vi "WS1050 16 DUT VSA-CV Sweep HD_Cycling_Ver1.3.vi"() -> ()   [LabVIEW 2012]
uses:
  WS_VCAP Driver 024/Source/WSVCAP Shell/Type Defs/WSVCAP SHL I2C DUT Mask Mode Enum.ctl
  <vilib>/Utility/file.llb/Read From Spreadsheet File (DBL).vi
panel:
  out "VISA resource name out":refnum<visa-resource-name>="GPIB0::3::INSTR"
  out "date string":string="5/19/2014"
  out "PS1 Out":refnum<visa-resource-name>
  out "Ke2000 Out":refnum<visa-resource-name>="GPIB0::9::INSTR"
  in  "Tab Control":enum32{"Inst Control", "Data Output", "Graphs"}(tab)
  in  "Bank to HD":u16(ring)=5 items=["All OFF", "All ON", "Bank_C1", "Bank_C2", "Bank_C3", "F12+B1"]
  out "AD7747 Values":string[][](table)
  in  "Lot#":string="4NEMB"
  in  "Wafer#":string="20-EB"
  in  "File Name":string="HD_4NEMB_25_EB_65C_44V_100DC_BRD2_150916_1"
  in  "TMN DC\\CAP Data Log File Path":path=path "C:/WS1050 16 DUT Data"
  in  "SN":string[](array[string])=["1", "2", "3", "4", "5", "6", "7", "8", "9", "10", "11", "12", "13", "14", "15", "16"]
  in  "Test Program":string="WS1050 16 DUT VSA_CV Sweep HD_Cycling Ver1.3"
  out "Current Date":string="8/28/2014"
  out "Current Time":string="0950"
  in  "Start Date":string="4/24/2014"
  in  "Start Time":string="1542"
  in  "Comment":string="CV Sweep"
  in  "OK Button":bool
  in  "Calibration":bool
  in  "Control Setting":bool
  in  "CP Setting":i32(ring) items=["CP OFF", "CP ON", "CP 35V", "CP 40V", "CP 44V", "CP 50V", "DVA OFF", "DVA ON", "Reg1 ON", "Reg1 OFF", "Reg2 ON", "Reg2 OFF", "Reg3 ON", "Reg3 OFF"]
  in  "VDD(V)":dbl=3.3 format="%.3g"
  in  "Meas Clock Rate (Hz)":dbl=1000000.0 caption="Meas Speed" format="%.1p Hz"
  out "AR  Measurent(Hz)":dbl
  in  "PS1 Source":refnum<visa-resource-name>="GPIB0::5::INSTR"
  in  "Ke2000":refnum<visa-resource-name>="GPIB0::9::INSTR"
  out "Simulate FPGA":bool
  out "Online":bool
  in  "Ke2400":refnum<visa-resource-name>="GPIB0::3::INSTR"
  in  "Initialize AD7747":bool
  in  "DUT Mask Mode":T1=enum."All"
  in  "RFFE Slave Address":u8=7 caption="Slave Address" format="0x%02x"
  out "Activity Log":string="05/19/2014 -- 12:24:35.853::WSVCAP::APP::Application Started\n05/19/2014 -- 12:24:37.606::WSVCAP::WSVCAP SHL::WR I2C-REG:0x0A;MASK:0xFFFFFFFFFFFF;C1 DATA:22:22:22:22:22:22:22:22:22:22:22:22:22:22:22:22;C2 DATA:22:22:22:22:22:22:22:22:22:22:22:22:22:22:22:22;C3 DATA:22:22:22:22:22:22:22:22:22:22:22:22:22:22:22:22\r\n05/19/2014 -- 12:24:37.773::WSVCAP::WSVCAP SHL::WR I2C-ST:0,0,4,1\r\n05/19/2014 -- 12:24:37.903::WSVCAP::WSVCAP SHL::RD I2C-BYTES:4;ADD:0x00;MASK:0xFFFFFFFFFFFF\r\n05/19/2014 -- 12:24:38.045::WSVCAP::WSVCAP SHL::RD I2C:C1 DATA:2:2:2:2:2:2:2:2:2:2:2:2:2:2:2:2|A7:A9:AA:82:82:7F:82:81:82:81:83:82:81:82:82:81|46:36:BB:88:44:A3:E9:2B:32:20:ED:25:BB:3D:68:B|2C:6A:EB:A7:22:56:FE:CC:36:82:D7:B0:3B:48:F9:CC;C2 DATA:2:2:2:2:2:2:2:2:2:2:2:2:2:2:2:2|94:94:94:80:80:80:80:80:81:7E:7E:81:80:7E:80:80|47:33:15:82:62:B:E8:1C:D7:C3:7D:41:7C:B7:4C:2A|C4:B4:AE:8:1E:D1:4E:37:11:C0:6F:63:42:9D:63:B5;C3 DATA:2:2:2:2:2:2:2:2:2:2:2:2:2:2:2:2|95:95:95:81:81:7E:81:80:84:7D:80:83:81:7E:7F:80|AB:C4:14:B5:7B:52:DF:C9:79:5D:5F:30:99:31:1E:F4|6E:5C:F7:A8:C3:EB:7B:EF:33:92:89:77:4D:67:75:DD;STATUS:0:0:4:0\r\n05/19/2014 -- 12:24:38.046::WSVCAP::WSVCAP SHL::WR I2C-REG:0x0A;MASK:0xFFFFFFFFFFFF;C1 DATA:22:22:22:22:22:22:22:22:22:22:22:22:22:22:22:22;C2 DATA:22:22:22:22:22:22:22:22:22:22:22:22:22:22:22:22;C3 DATA:22:22:22:22:22:22:22:22:22:22:22:22:22:22:22:22\r\n05/19/2014 -- 12:24:38.089::WSVCAP::WSVCAP SHL::WR I2C-ST:0,0,4,1\r\n05/19/2014 -- 12:24:38.219::WSVCAP::WSVCAP SHL::RD I2C-BYTES:4;ADD:0x00;MASK:0xFFFFFFFFFFFF\r\n05/19/2014 -- 12:24:38.362::WSVCAP::WSVCAP SHL::RD I2C:C1 DATA:2:2:2:2:2:2:2:2:2:2:2:2:2:2:2:2|A7:AB:AA:82:82:82:83:83:82:82:82:82:7F:82:82:81|4B:32:96:83:3E:61:43:17:25:62:AB:4D:A2:40:2E:5|3C:76:2B:B4:EE:E4:A9:1A:AA:A:26:C7:21:2E:87:5B;C2 DATA:2:2:2:2:2:2:2:2:2:2:2:2:2:2:2:2|94:94:94:80:80:80:80:80:80:7F:80:81:80:80:7F:80|4A:32:19:7D:19:6C:79:46:61:7F:4B:B8:A5:30:F3:14|B4:70:A:8C:9C:DC:43:FA:1E:A:C6:21:A:A9:13:F3;C3 DATA:2:2:2:2:2:2:2:2:2:2:2:2:2:2:2:2|95:97:94:81:80:81:82:81:80:7E:81:84:7F:81:80:80|B2:32:D0:A7:9E:4C:AB:D4:EE:D9:F0:82:B7:91:7:FF|C1:91:B6:3D:D8:E:1B:4F:9F:6A:F1:6C:E7:3F:7:BA;STATUS:0:0:4:0\r\n05/19/2014 -- 12:24:38.364::WSVCAP::WSVCAP SHL::WR I2C-REG:0x0A;MASK:0xFFFFFFFFFFFF;C1 DATA:22:22:22:22:22:22:22:22:22:22:22:22:22:22:22:22;C2 DATA:22:22:22:22:22:22:22:22:22:22:22:22:22:22:22:22;C3 DATA:22:22:22:22:22:22:22:22:22:22:22:22:22:22:22:22\r\n05/19/2014 -- 12:24:38.406::WSVCAP::WSVCAP SHL::WR I2C-ST:0,0,4,1\r\n05/19/2014 -- 12:24:38.536::WSVCAP::WSVCAP SHL::RD I2C-BYTES:4;ADD:0x00;MASK:0xFFFFFFFFFFFF\r\n05/19/2014 -- 12:24:38.678::WSVCAP::WSVCAP SHL::RD I2C:C1 DATA:2:2:2:2:2:2:2:2:2:2:2:2:2:2:2:2|A7:A9:AB:82:82:81:82:82:82:82:82:82:82:82:82:81|46:71:4C:87:43:3D:7F:FC:25:4F:8E:54:97:3E:60:8C|AA:F4:1F:B5:CE:43:1F:36:9:87:9C:78:86:5:B6:8E;C2 DATA:2:2:2:2:2:2:2:2:2:2:2:2:2:2:2:2|94:94:94:80:7F:7F:80:80:80:80:80:81:80:80:80:80|49:36:18:7D:6E:C5:E4:3C:81:2E:41:D3:75:71:E3:72|E8:D3:E6:D1:E0:48:AE:D4:54:D:E8:8E:B4:41:68:4;C3 DATA:2:2:2:2:2:2:2:2:2:2:2:2:2:2:2:2|95:95:95:81:7F:7F:81:81:81:81:81:84:81:81:82:81|B3:F5:90:AB:82:69:7B:93:D0:77:E8:D5:E8:8C:84:E8|B9:AC:EE:2B:B6:71:8F:4A:74:31:56:BB:8A:B7:A0:C8;STATUS:0:0:4:0\r\n05/19/2014 -- 12:24:38.681::WSVCAP::WSVCAP SHL::WR I2C-REG:0x0A;MASK:0xFFFFFFFFFFFF;C1 DATA:22:22:22:22:22:22:22:22:22:22:22:22:22:22:22:22;C2 DATA:22:22:22:22:22:22:22:22:22:22:22:22:22:22:22:22;C3 DATA:22:22:22:22:22:22:22:22:22:22:22:22:22:22:22:22\r\n05/19/2014 -- 12:24:38.723::WSVCAP::WSVCAP SHL::WR I2C-ST:0,0,4,1\r\n05/19/2014 -- 12:24:38.854::WSVCAP::WSVCAP SHL::RD I2C-BYTES:4;ADD:0x00;MASK:0xFFFFFFFFFFFF\r\n05/19/2014 -- 12:24:38.996::WSVCAP::WSVCAP SHL::RD I2C:C1 DATA:2:2:2:2:2:2:2:2:2:2:2:2:2:2:2:2|A7:A9:AA:82:82:7F:83:81:82:81:84:82:7F:82:7F:82|43:FB:E:7F:3C:AD:35:35:26:A2:6C:21:4B:3D:8:6|63:9A:E1:F3:95:32:91:42:90:3C:78:1F:5C:D7:5F:D8;C2 DATA:2:2:2:2:2:2:2:2:2:2:2:2:2:2:2:2|94:94:94:80:80:80:80:80:81:80:7E:81:80:7E:7F:80|48:36:18:7F:5E:3D:69:83:DE:AE:A1:9E:31:AE:BB:96|15:A0:44:17:13:FD:CC:C8:6D:B2:EF:A7:C:C7:3B:F;C3 DATA:2:2:2:2:2:2:2:2:2:2:2:2:2:2:2:2|95:96:94:81:81:7E:82:80:84:80:80:84:7F:7E:7D:82|AD:3B:6D:A9:7C:57:9D:F5:7A:96:23:5C:36:2D:ED:5A|CD:46:DB:3B:C7:BD:70:60:33:B8:B:F7:63:A:51:4D;STATUS:0:0:4:0\r\n05/19/2014 -- 12:24:38.998::WSVCAP::WSVCAP SHL::WR I2C-REG:0x0A;MASK:0xFFFFFFFFFFFF;C1 DATA:22:22:22:22:22:22:22:22:22:22:22:22:22:22:22:22;C2 DATA:22:22:22:22:22:22:22:22:22:22:22:22:22:22:22:22;C3 DATA:22:22:22:22:22:22:22:22:22:22:22:22:22:22:22:22\r\n05/19/2014 -- 12:24:39.040::WSVCAP::WSVCAP SHL::WR I2C-ST:0,0,4,1\r\n05/19/2014 -- 12:24:39.170::WSVCAP::WSVCAP SHL::RD I2C-BYTES:4;ADD:0x00;MASK:0xFFFFFFFFFFFF\r\n05/19/2014 -- 12:24:39.311::WSVCAP::WSVCAP SHL::RD I2C:C1 DATA:2:2:2:2:2:2:2:2:2:2:2:2:2:2:2:2|A7:AA:AB:82:82:81:82:81:82:81:82:82:82:82:7F:82|44:F1:90:87:45:44:C8:2C:2C:F1:FC:1B:94:3B:3C:75|4A:49:95:19:99:73:64:3:23:24:F3:A2:5E:7F:C4:B6;C2 DATA:2:2:2:2:2:2:2:2:2:2:2:2:2:2:2:2|94:94:94:80:80:80:80:7F:80:80:7E:80:80:7E:7F:80|4C:36:17:7D:A8:9F:DE:C7:53:6D:8A:F4:41:A5:C6:E0|90:2E:24:C:D9:22:E4:76:3B:40:1D:53:33:B1:3E:4D;C3 DATA:2:2:2:2:2:2:2:2:2:2:2:2:2:2:2:2|95:97:95:81:81:7F:81:80:80:81:7F:82:81:7E:7D:82|AE:2B:A7:AB:CC:CD:A4:38:FD:17:80:F2:92:2D:45:C4|76:E5:D:B9:AD:B5:BA:8D:28:32:9E:42:B7:20:4A:D9;STATUS:0:0:4:0\r\n05/19/2014 -- 12:24:39.313::WSVCAP::WSVCAP SHL::WR I2C-REG:0x0A;MASK:0xFFFFFFFFFFFF;C1 DATA:22:22:22:22:22:22:22:22:22:22:22:22:22:22:22:22;C2 DATA:22:22:22:22:22:22:22:22:22:22:22:22:22:22:22:22;C3 DATA:22:22:22:22:22:22:22:22:22:22:22:22:22:22:22:22\r\n05/19/2014 -- 12:24:39.355::WSVCAP::WSVCAP SHL::WR I2C-ST:0,0,4,1\r\n05/19/2014 -- 12:24:39.486::WSVCAP::WSVCAP SHL::RD I2C-BYTES:4;ADD:0x00;MASK:0xFFFFFFFFFFFF\r\n05/19/2014 -- 12:24:39.628::WSVCAP::WSVCAP SHL::RD I2C:C1 DATA:2:2:2:2:2:2:2:2:2:2:2:2:2:2:2:2|A7:A9:AA:82:82:82:83:82:82:82:82:82:7F:82:7F:82|47:18:E4:87:3E:E7:6:65:25:92:37:38:A8:3E:89:85|7C:A7:7:2B:A3:7A:EC:EF:89:ED:F4:D3:D8:BC:3A:F5;C2 DATA:2:2:2:2:2:2:2:2:2:2:2:2:2:2:2:2|94:94:94:80:7F:80:80:7F:81:80:7E:80:80:80:81:80|49:37:17:80:76:25:6A:F8:DF:55:97:4D:B8:5B:2B:B1|13:E3:9A:3E:1A:2D:4F:B6:DB:E9:61:FA:8B:D6:9:CC;C3 DATA:2:2:2:2:2:2:2:2:2:2:2:2:2:2:2:2|95:95:95:81:7F:80:82:81:84:80:7F:81:80:81:7F:82|AF:93:3B:AF:5B:11:82:E4:7E:C3:2D:72:9:96:D9:A|DB:96:F2:10:5F:64:9A:C6:98:12:27:7D:10:D3:20:D9;STATUS:0:0:4:0\r\n05/19/2014 -- 12:24:40.132::WSVCAP::WSVCAP SHL::CLOSE\r\n"
  in  "C1 Cap DAC":u8=128 caption="B Data In" format="0x%02x"
  in  "C2 Cap DAC":u8=128 caption="B Data In" format="0x%02x"
  in  "C3 Cap DAC":u8=128 caption="B Data In" format="0x%02x"
  out "IDD Brd(uA)":string
  in  "VSA_IDD(A)":dbl=0.1
  in  "Stress Voltage(V)":dbl
  in  "Reset PS":bool
  in  "HD/Cycling":bool
  in  "Cyc Clock Rate (Hz)":dbl=5000000.0 caption="Cycle Speed" format="%.1p Hz"
  in  "Bank to Cycle":u16(ring)=1 items=["Cycle All", "Cycle F12+S1", "Cycle All - F12"]
  in  "Set Delay":dbl[](array[numeric])=[1.8e-05, 1.8e-05, 1.8e-05] min=0.0 max=0.5 format="%#.0p s"
  in  "CP Freq":u16(ring)=3 items=["000", "001", "010", "011", "100", "101", "110", "111"]
  in  "CP to HD/Cycle":i32(ring)=4 items=["CP HDC 35V", "CP HDC 40.25V", "CP HDC 27.5V", "CP HDC 30.5V", "CP HDC 44V", "CP HDC 50V"]
  in  "Cycle Freq(KHz)":dbl
  in  "RP will be\nFrom Lookup Table":bool
  out "STATUS":string="Idle...."
  in  "stop":bool
  out "C1 Min_T0":string[](array[string])
  out "CAP_Value(pF)":string[][](array[string])
  out "C3 Min_T0":string[](array[string])
  out "C2 Min_T0":string[](array[string])
  in  "Abort":bool
  out "error out 2":errorcluster
  in  "Set Stress to\nComplete(Cyc/Min)":u64=8100
  out "Verify Test Condition":string[](array[string])
  out "CMin+VCAP":string[][](table)
  out "Verify Drivers to Stress":string[](array[string])
  out "Cycle Count":u64 min=1 max=4 step=1
  out "Stress \nCompleted(Min)":u64
  out "Previous Time":string="12:20:26 PM"
  out "Delta CAP_T0(pF)":dbl[][](array[numeric])
  out "Delta CAP_Tc(pF)":dbl[][](array[numeric])
  in  "error in (no error)":errorcluster
  out "error out":errorcluster
  out "CP_IDD(uA)":string
  # "Company:  WiSpry Inc 20 Fairbanks \nSte 198 Irvine CA 92618\n\nAuthor:  Andy V Tran\nCreated:  01/13/2016\nLabVIEW 2012 Pro\nTP:  WS1050 16 DUT VSA_CV Sweep HD_Cycling Ver1.3\nFPGA Version: WS_VCAP Driver 024"
  # "Note:  Ver1.0 is a original version.\n\n1.  Two look up tables, \n      a.  1st is for Stress\n      b.  2nd is for Voltage sweep\n\nVer1.1\n\n1.  No Voltage to CAP Head for initial read point\n\nVer1.2\n\n1.  Add CP Freq\n\nVer1.3\n\n1.  Add Cycling Stress\n2.  Add a button for Readpoint from look up table\n3.  Add a selectable drivers for HD\n\nSet up and Test Sequences:\n\n1.  Calibration with Empty Sockets\n2.  Load Parts\n3.  Set condition to stress (CP Voltage, Drivers to Stress, CP to stress...)\n4.  Set Date/Time to start stressing\n5.  Set TTF to stop stressing (default = 135 hrs)"
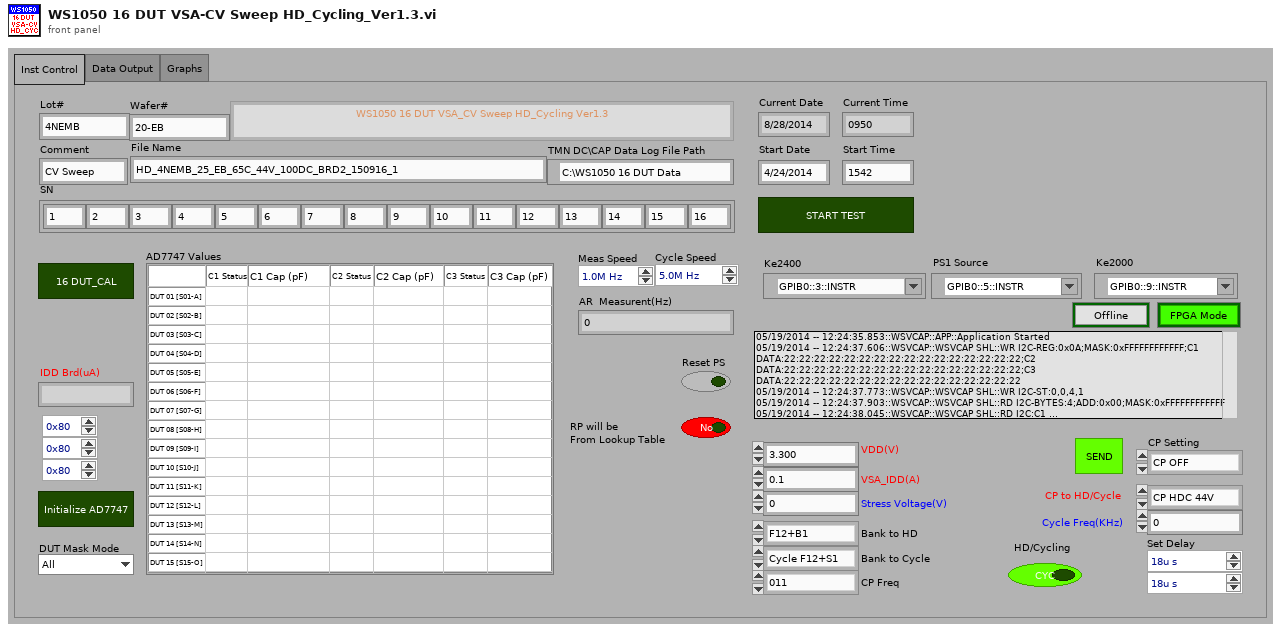
[diagram p1: front panel]
types:
  T1 = typedef "WSVCAP SHL I2C DUT Mask Mode Enum.ctl" = enum16{"Custom", "C1", "C2", "C3", "All"}
  T2 = typedef "WSVCAP SHL Core System Cluster.ctl" = cluster{"Settings":T3, "FPGA Resource":tag, "Online":bool, "I2C Wait Ticks":u32, "SPI Wait Ticks":u32, "RFFE Wait Ticks":u32}
  T3 = typedef "WSVCAP SHL I2C Settings Cluster.ctl" = cluster{"FPGA Resource Name":string, "I2C Slave Address":u8, "I2C Clock Rate (Hz)":dbl, "SPI Clock Rate (Hz)":dbl, "RFFE Slave Address":u8, "RFFE Clock Rate (Hz)":dbl, "Simulate FPGA":bool, "C1 Cap DAC Default":u8, "C2 Cap DAC Default":u8, "C3 Cap DAC Default":u8}
  T4 = enum16{"Idle...", "Voltage 1", "Voltage 2", "Voltage 3"}[]
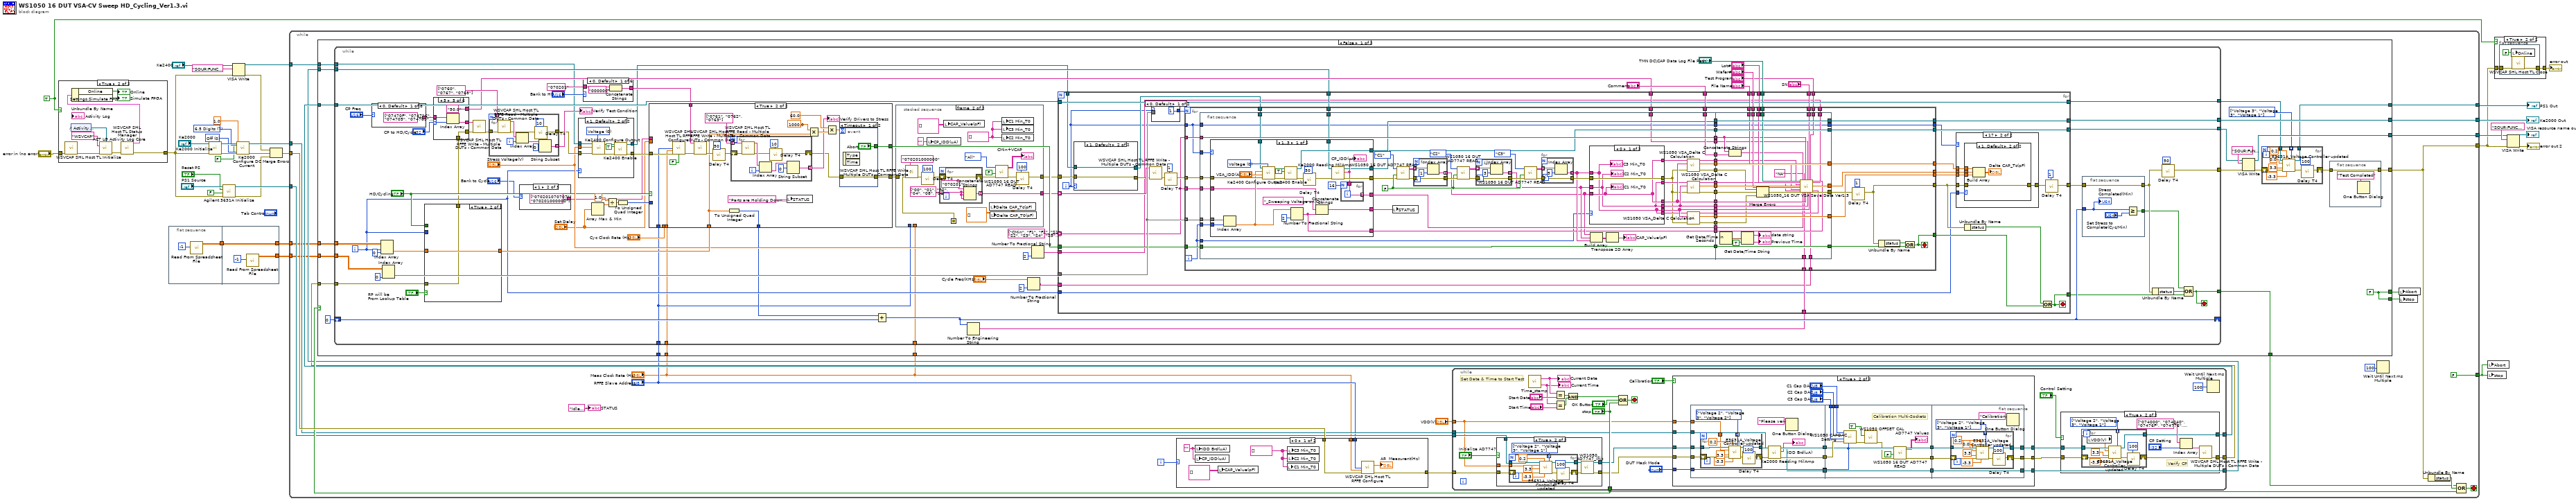
[diagram p0: block diagram]
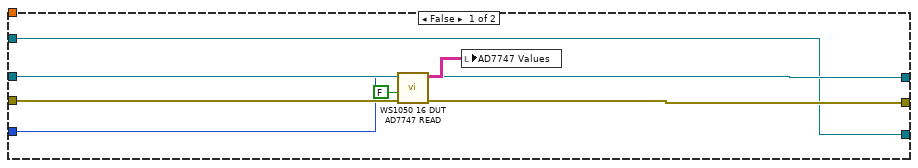
[diagram p7: hidden frame]
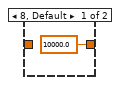
[diagram p9: hidden frame]
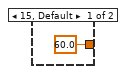
[diagram p11: hidden frame]
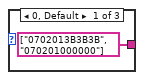
[diagram p12: hidden frame]
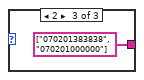
[diagram p13: hidden frame]
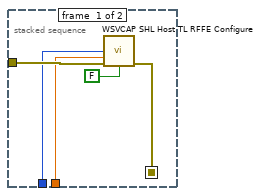
[diagram p14: hidden frame]
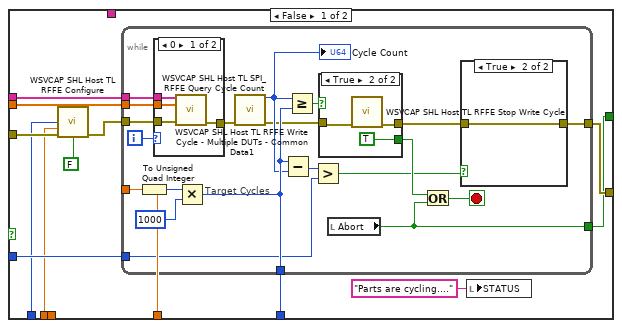
[diagram p15: hidden frame]
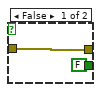
[diagram p18: hidden frame]
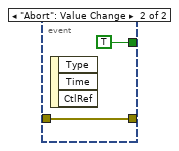
[diagram p19: hidden frame]
diagram:
  w21 = TRUE
  w27 = u16 0 items=["Off", "Moving Filter", "Repeating Filter"] ("Digital Filter (0: Off)")
  w28 = u16 7 items=["3.5 Digits"=4, "4.5 Digits"=5, "5.5 Digits"=6, "6.5 Digits"=7] ("Resolution (7: 6.5 digits)")
  n1 = case shown="True" w21 {
    tunnel: "error in (no error)" -> [w35 w36]
    tunnel: [w35 w43] -> w10
    frame False {
    }
    frame True {
      n2 = call "WSVCAP SHL Host TL Initialize.vi"("error in"=w36) -> ("error out"=w37:errorcluster)  [unwired: 13 in, 1 out]
      n3 = control-ref of="Activity Log"() -> (w39:refnum<vi>)
      n4 = call "ACT LG Activity Log Core.vi"("Display Ref"=w39, "Source"="WSVCAP", "Error In (no error)"=w37) -> ("Error Out"=w38:errorcluster)  [unwired: 11 in, 1 out]
      n5 = call "WSVCAP SHL Host TL Status Manager.vi"("error in"=w38) -> ("System Out"=w44:T2, "error out"=w43:errorcluster)  [unwired: 13 in]
      n6 = Unbundle By Name(w44) -> ("Online"=→"Online":bool, "Settings.Simulate FPGA"=→"Simulate FPGA":bool)
    }
  }
  n7 = flat-sequence {
    tunnel: [w46] -> w5
    tunnel: w5 -> [w49]
    tunnel: [w49] -> w4
    tunnel: [w48] -> w3
    frame #0 {
      n8 = call-poly <vilib>:"Read From Spreadsheet File.vi"("number of rows (all:-1)"=-1) -> ("all rows"=w46:dbl[][])  [unwired: 6 in, 4 out]
    }
    frame #1 {
      n9 = call-poly <vilib>:"Read From Spreadsheet File.vi"("number of rows (all:-1)"=-1) -> ("all rows"=w48:dbl[][])  [unwired: 6 in, 4 out]
    }
  }
  n10 = call "Ke2000 Initialize.vi"("error in (no error)"=w10, "VISA resource name"="Ke2000") -> ("error out"=w29:errorcluster, "VISA resource name out"=w30:refnum<visa-resource-name>)  [unwired: 8 in]
  n11 = call "Agilent 3631A Initialize.vi"("error in (no error)"=w10, "Default"=FALSE ("Reset? (T: Yes)"), "Reset"="Reset PS", "VISA resource name"="PS1 Source") -> ("error out"=w9:errorcluster, "VISA resource name out"=w33:refnum<visa-resource-name>)  [unwired: 6 in]
  n12 = VISA Write(VISA resource name="Ke2400", write buffer="SOUR:FUNC VOLT;VOLT:MODE FIX;RANG 100;LEV 0.0;:SENS:FUNC \"CURR\";CURR:PROT 60E-3;RANG 100E-3;:OUTP ON", error in (no error)=w10) -> (VISA resource name out=w18:refnum<visa-resource-name>, error out=w13:errorcluster)  [unwired: 1 out]
  n13 = call "Ke2000 Configure DC Current.vi"("Resolution (7: 6.5 digits)"=w28, "Digital Filter (0: Off)"=w27, "Auto Range? (T: Auto)"=FALSE, "error in"=w29, "Custom Range (0 A)"=1.0, "VISA resource name"=w30) -> ("error out"=w11:errorcluster, "VISA resource name out"=w25:refnum<visa-resource-name>)  [unwired: 4 in]
  n14 = Merge Errors(w13, w11, w9) -> (w19:errorcluster)
  n15 = while {
    tunnel: w19 -> [w70]
    tunnel: [w60] -> w15
    tunnel: w33 -> [w64]
    tunnel: w25 -> [w65]
    tunnel: [w73] -> w24
    tunnel: [w72] -> w23
    tunnel: w18 -> [w69]
    tunnel: [w68] -> w16
    tunnel: [FALSE] -> w8
    tunnel: w4 -> [w56]
    tunnel: w3 -> [w55]
    i -> [w71]
    stop <- w74 stop-if-true
    n16 = case shown="0" w71 {
      tunnel: w70 -> [w84 w85]
      tunnel: [w83 w85] -> w66
      tunnel: "RFFE Slave Address" -> [w81 _]
      tunnel: "Meas Clock Rate (Hz)" -> [w77 _]
      frame 0 {
        w80 = string[] []
        w78 = "" ("uA")
        n17 = local write "IDD Brd(uA)"(w78) -> ()
        n18 = local write "CP_IDD(uA)"(w78) -> ()
        n19 = local write "CAP_Value(pF)"(string[][] []) -> ()
        n20 = local write "C1 Min_T0"(w80) -> ()
        n21 = local write "C3 Min_T0"(w80) -> ()
        n22 = local write "C2 Min_T0"(w80) -> ()
        n23 = call "WSVCAP SHL Host TL RFFE Configure.vi"("RFFE Slave Address"=w81, "Clock Rate (Hz)"=w77, "error in"=w84) -> ("Actual Rate (Hz)"=→"AR  Measurent(Hz)":dbl, "error out"=w83:errorcluster)  [unwired: 11 in]
      }
      frame 1, Default {
      }
    }
    n24 = while {
      tunnel: ["stop"] -> w67
      tunnel: w66 -> [w97]
      tunnel: [w89] -> w61
      tunnel: w64 -> [w95]
      tunnel: w65 -> [w91]
      tunnel: [w92] -> w63
      tunnel: [w90] -> w62
      tunnel: "VDD(V)" -> [w87]
      stop <- w104 stop-if-true
      # "Set Date & Time to Start Test"
      n25 = case shown="True" "Initialize AD7747" {
        tunnel: w97 -> [w113 w119]
        tunnel: [w113 w115] -> w96
        tunnel: w95 -> [w112 w117]
        tunnel: [w112 w116] -> w94
        tunnel: w87 -> [_ w114]
        frame False {
        }
        frame True {
          w120 = T4 [enum."Voltage 2", enum."Voltage 3", enum."Voltage 1"] items=["Idle...", "Voltage 1", "Voltage 2", "Voltage 3"]
          n26 = for {
            tunnel: w117 -> [w130]
            tunnel: w120 -> [w128] mode=indexing
            tunnel: [w127] -> w116
            shift-right: [w124] -> w118
            shift-left: w119 -> [w131]
            tunnel: w114 -> [w122]
            n27 = call "E3631A_Voltage Controller updated.vi"("VISA resource name"=w130, "I_VDD(A)"=0.2, "Channel Controller"=w128, "Voltage 1"=w122, "Voltage 2"=3.3, "error in (no error)"=w131, "Voltage 3"=-3.3) -> ("VISA resource name out"=w127:refnum<visa-resource-name>, "error out"=w123:errorcluster)  [unwired: 7 in]
            n28 = call "Delay T4.vi"("milliseconds to wait"=u32 100, "error in (no error)"=w123) -> ("error out"=w124:errorcluster)  [unwired: 9 in]
          }
          n29 = call "WS1050_AD7747_Init.vi"("error in"=w118) -> ("error out"=w115:errorcluster)  [unwired: 10 in]
        }
      }
      n30 = call "Time_stamp.vi"() -> ("date/time string"=w109:string, "date string"=w111:string)  [unwired: 2 in]
      "Current Date" <- w111
      "Current Time" <- w109
      n31 = Equal?(x=w111, y="Start Date") -> (x = y?=w107:bool)
      n32 = Equal?(x=w109, y="Start Time") -> (x = y?=w106:bool)
      n33 = And(x=w107, y=w106) -> (x .and. y?=w103:bool)
      n34 = Compound Arithmetic op=OR(w103, "OK Button", "stop") -> (w104:bool)
      n35 = case shown="True" "Calibration" {
        tunnel: w96 -> [w158 w177]
        tunnel: [w157 w174] -> w88
        tunnel: w94 -> [w156 w173]
        tunnel: "DUT Mask Mode" -> [w155 w169]
        tunnel: [w156 w168] -> w93
        tunnel: w91 -> [w154 w164]
        tunnel: [w154 w161] -> w90
        tunnel: w87 -> [_ w160]
        frame False {
          n36 = call "WS1050 16 DUT AD7747 READ.vi"("error in"=w158, "Log (T)"=FALSE, "DUT Mask Mode (All)"=w155) -> ("error out"=w157:errorcluster, "AD7747 Values"=w159:string[][])  [unwired: 7 in]
          n37 = local write "AD7747 Values"(w159) -> ()
        }
        frame True {
          n38 = flat-sequence {
            tunnel: w177 -> [w187]
            tunnel: [w182] -> w176
            tunnel: w173 -> [w186]
            tunnel: [w185] -> w172
            tunnel: w169 -> [w184]
            tunnel: [w184] -> w170
            tunnel: w164 -> [w180]
            tunnel: [w179] -> w163
            tunnel: w160 -> [w178]
            tunnel: w176 -> [w213]
            tunnel: [w212] -> w175
            tunnel: w172 -> [w211]
            tunnel: [w211] -> w171
            tunnel: w170 -> [w210]
            tunnel: "C1 Cap DAC" -> [w206]
            tunnel: "C2 Cap DAC" -> [w205]
            tunnel: "C3 Cap DAC" -> [w204]
            tunnel: w163 -> [w203]
            tunnel: [w203] -> w162
            tunnel: w175 -> [w216]
            tunnel: [w219] -> w174
            tunnel: w171 -> [w218]
            tunnel: [w215] -> w168
            tunnel: w162 -> [w214]
            tunnel: [w214] -> w161
            frame #0 {
              w188 = T4 [enum."Voltage 2", enum."Voltage 3", enum."Voltage 2"] items=["Idle...", "Voltage 1", "Voltage 2", "Voltage 3"]
              n39 = for {
                tunnel: w186 -> [w199]
                tunnel: w188 -> [w196] mode=indexing
                tunnel: [w195] -> w185
                shift-right: [w193] -> w181
                shift-left: w187 -> [w200]
                tunnel: w178 -> [w190]
                n40 = call "E3631A_Voltage Controller updated.vi"("VISA resource name"=w199, "I_VDD(A)"=0.2, "Channel Controller"=w196, "Voltage 1"=w190, "Voltage 2"=3.3, "error in (no error)"=w200, "Voltage 3"=-3.3) -> ("VISA resource name out"=w195:refnum<visa-resource-name>, "error out"=w192:errorcluster)  [unwired: 7 in]
                n41 = call "Delay T4.vi"("milliseconds to wait"=u32 100, "error in (no error)"=w192) -> ("error out"=w193:errorcluster)  [unwired: 9 in]
              }
              n42 = call "Ke2000 Reading MilAmp.vi"("error in (no error)"=w181, "VISA resource name"=w180) -> ("error out"=w182:errorcluster, "uA"=→"IDD Brd(uA)":string, "VISA resource name out"=w179:refnum<visa-resource-name>)  [unwired: 7 in]
              n43 = One Button Dialog(message="Please verify all sockets should be empty...") -> ()  [unwired: 1 in, 1 out]
            }
            frame #1 {
              # "Calibration Multi-Sockets"
              n44 = call "WS1050 CAPDAC Setting.vi"("DUT Mask Mode (All)"=w210, "error in"=w213, "C3 Cap DAC"=w204, "C2 Cap DAC"=w205, "C1 Cap DAC"=w206) -> ("error out"=w208:errorcluster)  [unwired: 5 in, 1 out]
              n45 = call "WS1050 OFFSET CAL.vi"("error in"=w208, "OFFSET CAL"=TRUE ("Read?")) -> ("error out"=w207:errorcluster)  [unwired: 8 in, 1 out]
              n46 = call "WS1050 16 DUT AD7747 READ.vi"("error in"=w207, "Log (T)"=FALSE, "DUT Mask Mode (All)"=w210) -> ("error out"=w212:errorcluster, "AD7747 Values"=→"AD7747 Values":string[][])  [unwired: 7 in]
            }
            frame #2 {
              w217 = T4 [enum."Voltage 2", enum."Voltage 3", enum."Voltage 1"] items=["Idle...", "Voltage 1", "Voltage 2", "Voltage 3"]
              n47 = for {
                tunnel: w218 -> [w231]
                tunnel: w217 -> [w227] mode=indexing
                tunnel: [w226] -> w215
                shift-right: [w222] -> w219
                shift-left: w216 -> [w228]
                n48 = call "E3631A_Voltage Controller updated.vi"("VISA resource name"=w231, "I_VDD(A)"=0.2, "Channel Controller"=w227, "Voltage 1"=0.0, "Voltage 2"=3.3, "error in (no error)"=w228, "Voltage 3"=-3.3) -> ("VISA resource name out"=w226:refnum<visa-resource-name>, "error out"=w221:errorcluster)  [unwired: 7 in]
                n49 = call "Delay T4.vi"("milliseconds to wait"=u32 100, "error in (no error)"=w221) -> ("error out"=w222:errorcluster)  [unwired: 9 in]
              }
              n50 = One Button Dialog(message="Calibration Completed....") -> ()  [unwired: 1 in, 1 out]
            }
          }
        }
      }
      n51 = case shown="True" "Control Setting" {
        tunnel: [w132 w135] -> w89
        tunnel: w93 -> [w133 w138]
        tunnel: [w133 w136] -> w92
        tunnel: w88 -> [w132 w134]
        frame False {
        }
        frame True {
          w139 = T4 [enum."Voltage 2", enum."Voltage 3", enum."Voltage 1"] items=["Idle...", "Voltage 1", "Voltage 2", "Voltage 3"]
          # "Verify CP"
          n52 = for {
            tunnel: w138 -> [w151]
            tunnel: w139 -> [w148] mode=indexing
            shift-right: [w145] -> w137
            shift-left: w134 -> [w152]
            tunnel: [w143] -> w136
            n53 = local read "VDD(V)"() -> (w147:dbl)
            n54 = call "E3631A_Voltage Controller updated.vi"("VISA resource name"=w151, "Channel Controller"=w148, "Voltage 1"=w147, "Voltage 2"=3.3, "error in (no error)"=w152, "Voltage 3"=-3.3) -> ("VISA resource name out"=w143:refnum<visa-resource-name>, "error out"=w146:errorcluster)  [unwired: 8 in]
            n55 = call "Delay T4.vi"("milliseconds to wait"=u32 100, "error in (no error)"=w146) -> ("error out"=w145:errorcluster)  [unwired: 9 in]
          }
          n56 = Index Array(array=string[] ["074000", "074040", "07476F", "074776", "07477B", "07477C", "074820", "074800", "07413B", "074100", "07423B", "074200", "07433B", "074300"], index="CP Setting") -> (element=w140:string)
          n57 = call "WSVCAP SHL Host TL RFFE Write - Multiple DUTs - Common Data.vi"("Data Out"=w140, "error in"=w137) -> ("error out"=w135:errorcluster)  [unwired: 13 in]
        }
      }
      n58 = Wait Until Next ms Multiple(millisecond multiple=u32 100) -> ()  [unwired: 1 out]
    }
    n59 = case shown="False" w67 {
      tunnel: w61 -> [w251 w834]
      tunnel: [w235 w834] -> w60
      tunnel: w63 -> [w249 w832]
      tunnel: w62 -> [w252 w833]
      tunnel: [w248 w833] -> w73
      tunnel: [w239 w832] -> w72
      tunnel: w69 -> [w254 w831]
      tunnel: [w250 w831] -> w68
      tunnel: [w247 w830] -> w58
      tunnel: [w247 w830] -> w57
      tunnel: w56 -> [w245 _]
      tunnel: w55 -> [w243 _]
      tunnel: [w238 w830] -> w53
      tunnel: "RFFE Slave Address" -> [w234 _]
      tunnel: "Meas Clock Rate (Hz)" -> [w233 _]
      tunnel: "Meas Clock Rate (Hz)" -> [w232 _]
      frame False {
        w242 = T4 [enum."Voltage 3", enum."Voltage 3", enum."Voltage 1"] items=["Idle...", "Voltage 1", "Voltage 2", "Voltage 3"]
        w247 = FALSE
        n60 = while {
          tunnel: w254 -> [w289]
          tunnel: w252 -> [w301]
          tunnel: w251 -> [w279]
          tunnel: w249 -> [w334]
          tunnel: [w333] -> w248
          tunnel: [w332] -> w240
          tunnel: [w331] -> w246
          tunnel: [w330] -> w237
          tunnel: w245 -> [w322]
          shift-right: [w315] -> _
          shift-left: u64 0 ("disabled index (col)") -> [w320]
          tunnel: w243 -> [w313]
          tunnel: [w297] -> w238
          tunnel: w234 -> [w274]
          tunnel: w233 -> [w277]
          tunnel: w232 -> [w273]
          i -> [w280]
          stop <- w297 stop-if-true
          n61 = case shown="0, Default" "CP Freq" {
            tunnel: [string[] ["07470F", "074716", "074705", "074709", "07471B", "07471C"] string[] ["07471F", "074736", "074715", "074719", "07473B", "07473C"] string[] ["07474F", "074756", "074745", "074749", "07475B", "07475C"] string[] ["07476F", "074776", "074765", "074769", "07477B", "07477C"] string[] ["07478F", "074796", "074785", "074789", "07479B", "07479C"] string[] ["0747AF", "0747B6", "0747A5", "0747A9", "0747BB", "0747BC"] string[] ["0747BF", "0747C6", "0747B5", "0747B9", "0747CB", "0747CC"] string[] ["0747EF", "0747F6", "0747E5", "0747E9", "0747FB", "0747FC"]] -> w293
            frame 0, Default {
            }
            frame 1 {
            }
            frame 2 {
            }
            frame 3 {
            }
            frame 4 {
            }
            frame 5 {
            }
            frame 6 {
            }
            frame 7 {
            }
          }
          n62 = Index Array(array=w322, index (row)=w280, index (col)=0 ("disabled index (col)")) -> (element=w304:dbl)
          n63 = Index Array(array=w313, index (col)=0 ("disabled index (col)")) -> (element=w312:dbl[])  [unwired: 1 in]
          n64 = case shown="True" "RP will be\nFrom Lookup Table" {
            tunnel: w304 -> [w345 w359]
            tunnel: [w344 w359] -> w303
            tunnel: "HD/Cycling" -> [w343 _]
            tunnel: w280 -> [w342 _]
            tunnel: w279 -> [w341 w358]
            tunnel: [w340 w358] -> w278
            frame False {
              n65 = case shown="False" w343 {
                tunnel: w345 -> [w348 w355]
                tunnel: [w349 w354] -> w344
                tunnel: w342 -> [w347 w353]
                tunnel: w341 -> [w346 w352]
                tunnel: [w346 w352] -> w340
                frame False {
                  n66 = case shown="0..7" w347 {
                    tunnel: w348 -> [_ w351]
                    tunnel: [10000.0 w351] -> w349
                    frame 8, Default {
                    }
                    frame 0..7 {
                    }
                  }
                }
                frame True {
                  n67 = case shown="0..14" w353 {
                    tunnel: w355 -> [_ w357]
                    tunnel: [60.0 w357] -> w354
                    frame 15, Default {
                    }
                    frame 0..14 {
                    }
                  }
                }
              }
            }
            frame True {
            }
          }
          n68 = case shown="5" "CP to HD/Cycle" {
            selector: "CP to HD/Cycle" -> [w524 w529 w534 w539 w544 w548]
            tunnel: w293 -> [w525 w530 w535 w540 w545 w550]
            tunnel: [w523 w528 w533 w538 w543 w549] -> w327
            tunnel: ["35.0" ("Data Out") "27.5" ("Data Out") "30.5" ("Data Out") "44.0" ("Data Out") "50.0" ("Data Out") "40.25" ("Data Out")] -> w308
            tunnel: [w521 w526 w531 w536 w541 w546] -> w326
            tunnel: w278 -> [w521 w526 w531 w536 w541 w546]
            frame 0, Default {
              n69 = Index Array(array=w525, index=w524) -> (element=w523:string)
            }
            frame 2 {
              n70 = Index Array(array=w530, index=w529) -> (element=w528:string)
            }
            frame 3 {
              n71 = Index Array(array=w535, index=w534) -> (element=w533:string)
            }
            frame 4 {
              n72 = Index Array(array=w540, index=w539) -> (element=w538:string)
            }
            frame 5 {
              n73 = Index Array(array=w545, index=w544) -> (element=w543:string)
            }
            frame 1 {
              n74 = Index Array(array=w550, index=w548) -> (element=w549:string)
            }
          }
          n75 = call "WSVCAP SHL Host TL RFFE Write - Multiple DUTs - Common Data.vi"("Data Out"=w327, "error in"=w326) -> ("error out"=w324:errorcluster)  [unwired: 13 in]
          n76 = for {
            tunnel: string[] ["0760", "0767", "0768"] -> [w520] mode=indexing
            tunnel: [w516] -> w323 mode=indexing
            tunnel: w324 -> [w514]
            tunnel: [w512] -> w290
            i -> [w519]
            n77 = call "WSVCAP SHL Host TL RFFE Read - Multiple DUTs - Common Data.vi"("Data Out"=w520, "error in"=w514) -> ("RFFE Data In"=w518:string[], "error out"=w511:errorcluster)  [unwired: 12 in]
            n78 = Index Array(array=w518, index=w519) -> (element=w515:string)
            n79 = call "Delay T4.vi"("milliseconds to wait"=u32 10, "error in (no error)"=w511) -> ("error out"=w512:errorcluster)  [unwired: 9 in]
            n80 = String Subset(string=w515, offset (0)=0) -> (substring=w516:string)  [unwired: 1 in]
          }
          "Verify Test Condition" <- w323
          n81 = case shown="1" "Bank to Cycle" {
            tunnel: [string[] ["0702013B3B3B", "070201000000"] ("Command 2") string[] ["070201070707", "070201000000"] ("Command 2") string[] ["070201383838", "070201000000"] ("Command 2")] -> w271
            frame 0, Default {
            }
            frame 1 {
            }
            frame 2 {
            }
          }
          n82 = case shown="1, Default" w280 {
            tunnel: [w470 w477] -> w287
            tunnel: w290 -> [w470 w476]
            tunnel: w289 -> [w471 w475]
            tunnel: [w471 w474] -> w288
            tunnel: "Stress Voltage(V)" -> [_ w472]
            frame 0 {
            }
            frame 1, Default {
              w473 = u16 0 items=["Voltage", "Current"] ("Source Mode  (0: Voltage)")
              n83 = call "Ke2400 Configure Output.vi"("Source Mode  (0: Voltage)"=w473, "error in (no error)"=w476, "Output Level (0)"=w472, "VISA resource name"=w475) -> ("error out"=w480:errorcluster, "VISA resource name out"=w478:refnum<visa-resource-name>)  [unwired: 6 in]
              n84 = call "Ke2400 Enable.vi"("error in (no error)"=w480, "ON/OFF"=TRUE ("Enable Output (T: Enable)"), "VISA resource name"=w478) -> ("error out"=w477:errorcluster, "VISA resource name out"=w474:refnum<visa-resource-name>)  [unwired: 7 in]
            }
          }
          n85 = case shown="0, Default" "Bank to HD" {
            tunnel: "070201" -> [w491 w493 w496 w499 w502 w505]
            tunnel: [w489 w492 w495 w498 w501 w504] -> w294
            frame 0, Default {
              n86 = Concatenate Strings(w491, "000000" ("string")) -> (w489:string)
            }
            frame 1 {
              n87 = Concatenate Strings(w493, "3B3B3B" ("string")) -> (w492:string)
            }
            frame 2 {
              n88 = Concatenate Strings(w496, "3B0000" ("string")) -> (w495:string)
            }
            frame 3 {
              n89 = Concatenate Strings(w499, "003B00" ("string")) -> (w498:string)
            }
            frame 4 {
              n90 = Concatenate Strings(w502, "00003B" ("string")) -> (w501:string)
            }
            frame 5 {
              n91 = Concatenate Strings(w505, "070707" ("string")) -> (w504:string)
            }
          }
          n92 = Array Max & Min(array="Set Delay") -> (max value=w284:dbl)  [unwired: 3 out]
          n93 = Divide(x=1.0, y=w284) -> (x/y=w283:dbl)
          n94 = To Unsigned Quad Integer(1:w283) -> (0:w282:u64)
          n95 = case shown="True" "HD/Cycling" {
            tunnel: [w397 w455] -> w311
            tunnel: w303 -> [w399 w442]
            tunnel: w294 -> [_ w454]
            tunnel: [w398 w453] -> w291
            tunnel: w287 -> [w394 w439]
            tunnel: w271 -> [w402 _]
            tunnel: "Set Delay" -> [w401 _]
            tunnel: w282 -> [w400 _]
            tunnel: [w396 w441] -> w276
            tunnel: "Cyc Clock Rate (Hz)" -> [w392 _]
            tunnel: w274 -> [w391 w436]
            tunnel: w273 -> [_ w435]
            frame False {
              n96 = call "WSVCAP SHL Host TL RFFE Configure.vi"("RFFE Slave Address"=w391, "Clock Rate (Hz)"=w392, "error in"=w394, "Log (T)"=FALSE) -> ("error out"=w393:errorcluster)  [unwired: 10 in, 1 out]
              n97 = while {
                tunnel: w399 -> [w422]
                tunnel: [w412] -> w398
                tunnel: [w407] -> w397
                tunnel: w393 -> [w420]
                tunnel: [w411] -> w396
                tunnel: w402 -> [w419]
                tunnel: w401 -> [w418]
                tunnel: w400 -> [w409]
                i -> [w417]
                stop <- w415 stop-if-true
                # "Target Cycles"
                n98 = To Unsigned Quad Integer(1:w422) -> (0:w421:u64)
                n99 = case shown="0" w417 {
                  tunnel: [w428 w429] -> w405
                  tunnel: w420 -> [w427 w429]
                  tunnel: w419 -> [w426 _]
                  tunnel: w418 -> [w425 _]
                  frame 0 {
                    n100 = call "WSVCAP SHL Host TL RFFE Write Cycle - Multiple DUTs - Common Data1.vi"("Data Out (Cycle Commands)"=w426, "Post Command Delay"=w425, "error in"=w427) -> ("error out"=w428:errorcluster)  [unwired: 12 in]
                  }
                  frame 1, Default {
                  }
                }
                n101 = Multiply(x=w421, y=u64 1000) -> (x*y=w411:u64)
                n102 = call "WSVCAP SHL Host TL SPI_RFFE Query Cycle Count.vi"("error in"=w405) -> ("Cycle Count"=w404:u64, "error out"=w403:errorcluster)  [unwired: 13 in]
                "Cycle Count" <- w404
                n103 = Subtract(x=w411, y=w404) -> (x-y=w410:u64)
                n104 = Greater Or Equal?(x=w404, y=w411) -> (x >= y?=w416:bool)
                n105 = Greater?(x=w410, y=w409) -> (0:w408:bool)
                n106 = case shown="True" w416 {
                  tunnel: [w431 w433] -> w413
                  tunnel: w403 -> [w431 w432]
                  tunnel: [FALSE TRUE] -> w414
                  frame False {
                  }
                  frame True {
                    n107 = call "WSVCAP SHL Host TL RFFE Stop Write Cycle.vi"("error in"=w432) -> ("error out"=w433:errorcluster)  [unwired: 14 in]
                  }
                }
                n108 = local read "Abort"() -> (w407:bool)
                n109 = Or(x=w414, y=w407) -> (x .or. y?=w415:bool)
                n110 = case shown="True" w408 {
                  tunnel: w413 -> [w423 w424]
                  tunnel: [w423 w424] -> w412
                  frame False {
                  }
                  frame True {
                  }
                }
              }
              n111 = local write "STATUS"("Parts are cycling...." ("STATUS")) -> ()
            }
            frame True {
              n112 = call "WSVCAP SHL Host TL RFFE Configure.vi"("RFFE Slave Address"=w436, "Clock Rate (Hz)"=w435, "error in"=w439, "Log (T)"=FALSE) -> ("error out"=w438:errorcluster)  [unwired: 10 in, 1 out]
              n113 = call "WSVCAP SHL Host TL RFFE Write - Multiple DUTs - Common Data.vi"("Data Out"=w454, "error in"=w438) -> ("error out"=w448:errorcluster)  [unwired: 13 in]
              n114 = call "Delay T4.vi"("milliseconds to wait"=u32 50, "error in (no error)"=w448) -> ("error out"=w445:errorcluster)  [unwired: 9 in]
              n115 = To Unsigned Quad Integer(1:w442) -> (0:w441:u64)
              n116 = for {
                tunnel: string[] ["0761", "0762", "0763"] -> [w465] mode=indexing
                tunnel: [w461] -> w444 mode=indexing
                shift-right: [w458] -> w443
                shift-left: w445 -> [w464]
                i -> [w463]
                n117 = call "WSVCAP SHL Host TL RFFE Read - Multiple DUTs - Common Data.vi"("Data Out"=w465, "error in"=w464) -> ("RFFE Data In"=w460:string[], "error out"=w457:errorcluster)  [unwired: 12 in]
                n118 = Index Array(array=w460, index=w463) -> (element=w459:string)
                n119 = call "Delay T4.vi"("milliseconds to wait"=u32 10, "error in (no error)"=w457) -> ("error out"=w458:errorcluster)  [unwired: 9 in]
                n120 = String Subset(string=w459, offset (0)=0) -> (substring=w461:string)  [unwired: 1 in]
              }
              "Verify Drivers to Stress" <- w444
              n121 = local write "STATUS"("Parts are Holding Down...." ("STATUS")) -> ()
              n122 = Multiply(x=1000.0, y=w442) -> (x*y=w451:dbl)
              n123 = Multiply(x=60.0, y=w451) -> (x*y=w452:dbl)
              n124 = event shown="[0] Timeout" {
                selector: _ -> [_ _]
                dyn-events: _ -> [_ _]
                timeout: w452 -> [_ _]
                tunnel: ["Abort" TRUE ("Abort")] -> w455
                tunnel: w443 -> [w466 w468]
                tunnel: [w466 w468] -> w453
                event Timeout {
                  n125 = event-data() -> ()  [unwired: 1 in, 2 out]
                }
                event "Abort": Value Change {
                  n126 = event-data() -> ()  [unwired: 1 in, 3 out]
                }
              }
            }
          }
          n127 = Add(x=w276, y=w320) -> (x+y=w315:u64)
          n128 = stacked-sequence {
            seq-local: [w363 _] -> [_ w369]
            tunnel: [_ w385] -> w307
            tunnel: [_ w384] -> w302
            tunnel: w291 -> [w367 _]
            tunnel: w274 -> [w366 _]
            tunnel: w277 -> [w365 _]
            frame #0 {
              n129 = call "WSVCAP SHL Host TL RFFE Configure.vi"("RFFE Slave Address"=w366, "Clock Rate (Hz)"=w365, "error in"=w367, "Log (T)"=FALSE) -> ("error out"=w363:errorcluster)  [unwired: 10 in, 1 out]
            }
            frame #1 {
              w368 = dbl[][] [] ("Delta CAP_T0(pF)")
              w380 = string[] [] ("CP Current(uA)")
              n130 = call "WSVCAP SHL Host TL RFFE Write - Multiple DUTs - Common Data.vi"("Data Out"="070201000000", "error in"=w369) -> ("error out"=w376:errorcluster)  [unwired: 13 in]
              n131 = call "Delay T4.vi"("milliseconds to wait"=u32 100, "error in (no error)"=w376) -> ("error out"=w377:errorcluster)  [unwired: 9 in]
              n132 = local write "CP_IDD(uA)"("" ("CP_IDD(uA)")) -> ()
              n133 = for {
                tunnel: string[] ["00", "01", "02", "04", "08", "0C", "10", "14", "18", "1C", "20", "24", "28", "2C", "30", "34", "38", "3B", "00"] -> [w388] mode=indexing
                tunnel: [w387] -> w384 mode=indexing
                shift-right: [w386] -> w381
                shift-left: w377 -> [w386]
                n134 = Concatenate Strings("070201" ("string"), w388, w388, w388) -> (w387:string)
              }
              n135 = local write "CAP_Value(pF)"(string[][] [] ("VSA_Value(pF)")) -> ()
              n136 = local write "Delta CAP_Tc(pF)"(w368) -> ()
              n137 = local write "Delta CAP_T0(pF)"(w368) -> ()
              n138 = call "WS1050 16 DUT AD7747 READ.vi"("error in"=w381, "Log (T)"=FALSE, "DUT Mask Mode (All)"=WSVCAP_SHL_I2C_DUT_Mask_Mode_Enum."All") -> ("error out"=w373:errorcluster, "AD7747 Values"=→"CMin+VCAP":string[][])  [unwired: 7 in]
              n139 = local write "C1 Min_T0"(w380) -> ()
              n140 = local write "C3 Min_T0"(w380) -> ()
              n141 = local write "C2 Min_T0"(w380) -> ()
              n142 = call "Delay T4.vi"("milliseconds to wait"=u32 100, "error in (no error)"=w373) -> ("error out"=w385:errorcluster)  [unwired: 9 in]
            }
          }
          n143 = Number To Engineering String(4:w315) -> (0:w309:string)  [unwired: 3 in]
          n144 = Number To Fractional String(number="Cycle Freq(KHz)", precision (6)=i16 2) -> (F-format string=w267:string)  [unwired: 2 in]
          n145 = Number To Fractional String(number="Stress Voltage(V)", precision (6)=i16 2) -> (F-format string=w299:string)  [unwired: 2 in]
          n146 = for {
            tunnel: w307 -> [w566]
            tunnel: [w590] -> w331
            tunnel: [w573] -> w318
            tunnel: "Comment" -> [w588]
            tunnel: "Lot#" -> [w587]
            tunnel: "Wafer#" -> [w586]
            tunnel: "SN" -> [w585]
            tunnel: "File Name" -> [w584]
            tunnel: [w583] -> w332
            tunnel: w334 -> [w583]
            tunnel: [w582] -> w333
            tunnel: w312 -> [w579]
            tunnel: w311 -> [w578]
            tunnel: [w575] -> w310
            tunnel: w309 -> [w559]
            tunnel: w308 -> [w574]
            tunnel: "TMN DC\\CAP Data Log File Path" -> [w571]
            tunnel: "Test Program" -> [w570]
            tunnel: w288 -> [w564]
            tunnel: w302 -> [w568] mode=indexing
            tunnel: w301 -> [w563]
            tunnel: string[] ["CMin", "F1", "F2", "S1", "S2", "S3", "S4", "S5", "S6", "S7", "S8", "S9", "S10", "S11", "S12", "S13", "S14", "S14F12", "All OFF"] -> [w561] mode=indexing
            tunnel: w299 -> [w562]
            tunnel: w280 -> [w553]
            tunnel: w267 -> [w551]
            i -> [w560]
            stop <- w575 stop-if-true
            n147 = case shown="1, Default" w560 {
              tunnel: [w613 w623] -> w567
              tunnel: w566 -> [w620 w623]
              tunnel: [w619 w622] -> w565
              tunnel: w564 -> [w618 w622]
              frame 0 {
                w616 = u16 0 items=["Voltage", "Current"] ("Source Mode  (0: Voltage)")
                n148 = call "Ke2400 Configure Output.vi"("Source Mode  (0: Voltage)"=w616, "error in (no error)"=w620, "Output Level (0)"=0.0, "VISA resource name"=w618) -> ("error out"=w621:errorcluster, "VISA resource name out"=w614:refnum<visa-resource-name>)  [unwired: 6 in]
                n149 = call "Ke2400 Enable.vi"("error in (no error)"=w621, "ON/OFF"=TRUE ("Enable Output (T: Enable)"), "VISA resource name"=w614) -> ("error out"=w612:errorcluster, "VISA resource name out"=w619:refnum<visa-resource-name>)  [unwired: 7 in]
                n150 = call "Delay T4.vi"("milliseconds to wait"=u32 50, "error in (no error)"=w612) -> ("error out"=w613:errorcluster)  [unwired: 9 in]
              }
              frame 1, Default {
              }
            }
            n151 = call "WSVCAP SHL Host TL RFFE Write - Multiple DUTs - Common Data.vi"("Data Out"=w568, "error in"=w567) -> ("error out"=w569:errorcluster)  [unwired: 13 in]
            n152 = case shown="0, Default" w560 {
              tunnel: [1 w610] -> w589
              tunnel: w579 -> [_ w609]
              frame 0, Default {
              }
              frame 1..3 {
                n153 = Array Size(array=w609) -> (size(s)=w610:i32)
              }
            }
            n154 = call "Delay T4.vi"("milliseconds to wait"=u32 1, "error in (no error)"=w569) -> ("error out"=w581:errorcluster)  [unwired: 9 in]
            n155 = for {
              N: w589 -> [_]
              tunnel: w579 -> [w676]
              tunnel: w571 -> [w666]
              tunnel: [w675] -> w557
              tunnel: w581 -> [w674]
              tunnel: [w670] -> w590
              tunnel: w588 -> [w653]
              tunnel: w587 -> [w660]
              tunnel: w586 -> [w659]
              tunnel: w585 -> [w658]
              tunnel: w584 -> [w657]
              tunnel: w561 -> [w656]
              tunnel: [w651] -> w582
              tunnel: w565 -> [w643]
              tunnel: w578 -> [w642]
              tunnel: [w639] -> w576
              tunnel: w574 -> [w637]
              tunnel: w570 -> [w636]
              tunnel: w563 -> [w635]
              tunnel: w562 -> [w634]
              tunnel: w561 -> [w633]
              tunnel: w560 -> [w631]
              tunnel: w559 -> [w630]
              tunnel: [w628] -> w556
              tunnel: [w627] -> w555
              tunnel: [w626] -> w554
              tunnel: [w625] -> w552
              tunnel: w551 -> [w624]
              i -> [w629]
              stop <- w639 stop-if-true
              n156 = flat-sequence {
                tunnel: w676 -> [w728]
                tunnel: w629 -> [w727]
                tunnel: w674 -> [w729]
                tunnel: [w694] -> w671
                tunnel: [w708] -> w669
                tunnel: [w709] -> w668
                tunnel: [w710] -> w667
                tunnel: [w679] -> w665
                tunnel: [w711] -> w664
                tunnel: [w707] -> w663
                tunnel: [w706] -> w662
                tunnel: [w705] -> w661
                tunnel: w656 -> [w704]
                tunnel: [w704] -> w655
                tunnel: [w703] -> w654
                tunnel: w653 -> [w703]
                tunnel: [w702] -> w652
                tunnel: [w701] -> w649
                tunnel: [w700] -> w648
                tunnel: [w699] -> w647
                tunnel: [w689] -> w646
                tunnel: [w688] -> w645
                tunnel: [w687] -> w644
                tunnel: w643 -> [w686]
                tunnel: w642 -> [w685]
                tunnel: [w685] -> w641
                tunnel: [w684] -> w638
                tunnel: w637 -> [w684]
                tunnel: w631 -> [w682]
                tunnel: w635 -> [w681]
                tunnel: w633 -> [w680]
                tunnel: w631 -> [w678]
                tunnel: [w678] -> w632
                tunnel: w629 -> [w677]
                tunnel: [w825] -> w672
                tunnel: [w827] -> w670
                tunnel: [w826] -> w651
                tunnel: [w824] -> w628
                tunnel: [w823] -> w627
                tunnel: [w822] -> w626
                tunnel: w647 -> [w824]
                tunnel: w648 -> [w823]
                tunnel: w649 -> [w822]
                tunnel: w652 -> [w826]
                tunnel: w654 -> [w809]
                tunnel: w655 -> [w796]
                tunnel: w661 -> [w810]
                tunnel: w662 -> [w811]
                tunnel: w663 -> [w812]
                tunnel: w657 -> [w813]
                tunnel: w664 -> [w814]
                tunnel: w665 -> [w807]
                tunnel: w658 -> [w815]
                tunnel: w659 -> [w816]
                tunnel: w660 -> [w817]
                tunnel: w666 -> [w818]
                tunnel: w667 -> [w819]
                tunnel: w668 -> [w820]
                tunnel: w669 -> [w821]
                tunnel: w671 -> [w827]
                tunnel: w646 -> [w800]
                tunnel: w645 -> [w801]
                tunnel: w644 -> [w799]
                tunnel: w641 -> [w797]
                tunnel: [w797] -> w640
                tunnel: w638 -> [w795]
                tunnel: w636 -> [w794]
                tunnel: w634 -> [w793]
                tunnel: w632 -> [w792]
                tunnel: [w792] -> w625
                tunnel: w630 -> [w791]
                tunnel: w624 -> [w790]
                frame #0 {
                  w715 = FALSE ("Log (T)")
                  n157 = case shown="1..3" w682 {
                    tunnel: w729 -> [w754 w761]
                    tunnel: w728 -> [w753 _]
                    tunnel: w727 -> [w752 _]
                    tunnel: [w743 w761] -> w712
                    tunnel: [w741 w764] -> w711
                    tunnel: [w740 w759] -> w702
                    tunnel: [w739 w760] -> w694
                    tunnel: w686 -> [w737 w760]
                    tunnel: [w733 "0"] -> w679
                    tunnel: [w732 w756] -> w683
                    tunnel: w681 -> [w731 w759]
                    tunnel: w680 -> [w730 w757]
                    frame 1..3 {
                      w746 = u16 0 items=["Voltage", "Current"] ("Source Mode  (0: Voltage)")
                      n158 = Index Array(array=w753, index=w752) -> (element=w735:dbl)
                      n159 = call "Ke2400 Configure Output.vi"("Source Mode  (0: Voltage)"=w746, "error in (no error)"=w754, "Compliance  Level (0.1)"="VSA_IDD(A)", "Output Level (0)"=w735, "VISA resource name"=w737) -> ("error out"=w750:errorcluster, "VISA resource name out"=w748:refnum<visa-resource-name>)  [unwired: 5 in]
                      n160 = call "Ke2400 Enable.vi"("error in (no error)"=w750, "ON/OFF"=TRUE ("Enable Output (T: Enable)"), "VISA resource name"=w748) -> ("error out"=w751:errorcluster, "VISA resource name out"=w739:refnum<visa-resource-name>)  [unwired: 7 in]
                      n161 = Number To Fractional String(number=w735, precision (6)=i16 2) -> (F-format string=w733:string)  [unwired: 2 in]
                      n162 = call "Delay T4.vi"("milliseconds to wait"=u32 50, "error in (no error)"=w751) -> ("error out"=w738:errorcluster)  [unwired: 9 in]
                      n163 = Concatenate Strings(w730, "_Sweeping Voltage on CAP Head... ", w733) -> (w732:string)
                      n164 = call "Ke2000 Reading MilAmp.vi"("error in (no error)"=w738, "VISA resource name"=w731) -> ("error out"=w743:errorcluster, "uA"=w742:string, "VISA resource name out"=w740:refnum<visa-resource-name>)  [unwired: 7 in]
                      "CP_IDD(uA)" <- w742
                      n165 = for {
                        N: 16 -> [_]
                        tunnel: w742 -> [w755]
                        tunnel: [w755] -> w741 mode=indexing
                      }
                    }
                    frame 0, Default {
                      n166 = Concatenate Strings(w757, "_No Sweeping Voltage on CAP Head... ") -> (w756:string)
                      n167 = for {
                        N: 16 -> [_]
                        tunnel: "0" ("uA") -> [w766]
                        tunnel: [w766] -> w764 mode=indexing
                      }
                    }
                  }
                  n168 = local write "STATUS"(w683) -> ()
                  n169 = call "WS1050 16 DUT AD7747 READ.vi"("error in"=w712, "Log (T)"=w715, "DUT Mask Mode (All)"=WSVCAP_SHL_I2C_DUT_Mask_Mode_Enum."C1") -> ("error out"=w724:errorcluster, "AD7747 Values"=w726:string[][])  [unwired: 7 in]
                  n170 = for {
                    tunnel: w726 -> [w788] mode=indexing
                    tunnel: [w786] -> w695 mode=indexing
                    tunnel: w724 -> [w787]
                    tunnel: [w787] -> w723
                    n171 = Index Array(array=w788, index=1) -> (element=w786:string)
                  }
                  n172 = call "WS1050 16 DUT AD7747 READ.vi"("error in"=w723, "Log (T)"=w715, "DUT Mask Mode (All)"=WSVCAP_SHL_I2C_DUT_Mask_Mode_Enum."C2") -> ("error out"=w721:errorcluster, "AD7747 Values"=w720:string[][])  [unwired: 7 in]
                  n173 = for {
                    tunnel: w720 -> [w784] mode=indexing
                    tunnel: [w782] -> w696 mode=indexing
                    tunnel: w721 -> [w783]
                    tunnel: [w783] -> w719
                    n174 = Index Array(array=w784, index=3) -> (element=w782:string)
                  }
                  n175 = call "WS1050 16 DUT AD7747 READ.vi"("error in"=w719, "Log (T)"=w715, "DUT Mask Mode (All)"=WSVCAP_SHL_I2C_DUT_Mask_Mode_Enum."C3") -> ("error out"=w717:errorcluster, "AD7747 Values"=w716:string[][])  [unwired: 7 in]
                  n176 = for {
                    tunnel: w716 -> [w780] mode=indexing
                    tunnel: [w778] -> w713 mode=indexing
                    tunnel: w717 -> [w779]
                    tunnel: [w779] -> w714
                    n177 = Index Array(array=w780, index=5) -> (element=w778:string)
                  }
                  n178 = case shown="0" w677 {
                    tunnel: w714 -> [w770 w777]
                    tunnel: [w770 w777] -> w690
                    tunnel: w713 -> [w767 w774]
                    tunnel: w696 -> [w768 w775]
                    tunnel: w695 -> [w769 w776]
                    tunnel: [w769 w776] -> w708
                    tunnel: [w768 w775] -> w709
                    tunnel: [w767 w774] -> w710
                    tunnel: [w767 w773] -> w693
                    tunnel: [w768 w772] -> w692
                    tunnel: [w769 w771] -> w691
                    frame 0 {
                      "C3 Min_T0" <- w767
                      "C2 Min_T0" <- w768
                      "C1 Min_T0" <- w769
                    }
                    frame 1, Default {
                      n179 = local read "C3 Min_T0"() -> (w773:string[])
                      n180 = local read "C1 Min_T0"() -> (w771:string[])
                      n181 = local read "C2 Min_T0"() -> (w772:string[])
                    }
                  }
                  n182 = Build Array(w695, w696, w713) -> (w697:string[][])
                  n183 = Transpose 2D Array(2D array=w697) -> (transposed array=→"CAP_Value(pF)":string[][])
                  n184 = call "WS1050 VSA_Delta C Calculation.vi"("error in (no error)"=w690, "CAP_T"=w708, "CAP_T0"=w691) -> ("error out"=w689:errorcluster, 2:"Delta C(pF)"=w699:dbl[], 3:"Delta C(pF)"=w707:string[])  [unwired: 6 in]
                  n185 = call "WS1050 VSA_Delta C Calculation.vi"("error in (no error)"=w690, "CAP_T"=w709, "CAP_T0"=w692) -> ("error out"=w688:errorcluster, 2:"Delta C(pF)"=w700:dbl[], 3:"Delta C(pF)"=w706:string[])  [unwired: 6 in]
                  n186 = call "WS1050 VSA_Delta C Calculation.vi"("error in (no error)"=w690, "CAP_T"=w710, "CAP_T0"=w693) -> ("error out"=w687:errorcluster, 2:"Delta C(pF)"=w701:dbl[], 3:"Delta C(pF)"=w705:string[])  [unwired: 6 in]
                }
                frame #1 {
                  n187 = Get Date/Time In Seconds() -> (seconds since 1Jan1904=w806:timestamp)
                  n188 = Concatenate Strings(w796, w809) -> (w808:string)
                  n189 = Get Date/Time String(seconds (now)=w806, want seconds? (F)=TRUE) -> (date string=→"date string":string, time string=→"Previous Time":string)  [unwired: 1 in]
                  n190 = Merge Errors(w800, w801, w799) -> (w798:errorcluster)
                  n191 = call "WS1050_16 DUT VSA Save Data Ver1.3.vi"("TMN DC\\CAP Data Log File Path"=w818, "Lot#"=w817, "VSA_Delta C1(pF)"=w812, "Wafer#"=w816, "File Name"=w813, "VSA_Delta C2(pF)"=w811, "error in"=w798, "Comment"=w808, "CP Current(uA)"=w814, "VSA_IDD(A)"="NA", "HD Time(Min)"=w791, "Driver"=w796, "VSA_C1"=w821, "CP HD (V)"=w795, "VSA_C2"=w820, "SN"=w815, "VSA_C3"=w819, "Test Program"=w794, "Cyc_Freq(KHz)"=w790, "Voltage(V)"=w807, "Stress Voltage(V)"=w793, "VSA_Delta C3(pF)"=w810) -> ("error out"=w825:errorcluster)  [unwired: 5 in]
                }
              }
              n192 = call "Delay T4.vi"("milliseconds to wait"=u32 1, "error in (no error)"=w672) -> ("error out"=w675:errorcluster)  [unwired: 9 in]
              n193 = Unbundle By Name(w675) -> ("status"=w650:bool)
              n194 = Compound Arithmetic op=OR(w650, w640) -> (w639:bool)
            }
            n195 = case shown="17" w552 {
              tunnel: [w591 w597] -> w558
              tunnel: w557 -> [w591 w596]
              tunnel: w556 -> [_ w595]
              tunnel: w555 -> [_ w594]
              tunnel: w554 -> [_ w593]
              tunnel: w553 -> [_ w592]
              frame 0, Default {
              }
              frame 17 {
                n196 = case shown="1, Default" w592 {
                  tunnel: w595 -> [w601 w607]
                  tunnel: w594 -> [w600 w606]
                  tunnel: w593 -> [w599 w605]
                  tunnel: w596 -> [w598 w603]
                  tunnel: [w598 w603] -> w597
                  frame 0 {
                    n197 = Build Array(w601, w600, w599) -> (→"Delta CAP_T0(pF)":dbl[][])
                  }
                  frame 1, Default {
                    n198 = Build Array(w607, w606, w605) -> (→"Delta CAP_Tc(pF)":dbl[][])
                  }
                }
              }
            }
            n199 = Unbundle By Name(w557) -> ("status"=w577:bool)
            n200 = Or(x=w577, y=w576) -> (x .or. y?=w575:bool)
            n201 = call "Delay T4.vi"("milliseconds to wait"=u32 1, "error in (no error)"=w558) -> ("error out"=w573:errorcluster)  [unwired: 9 in]
          }
          n202 = flat-sequence {
            tunnel: w318 -> [w509]
            tunnel: [w509] -> w317
            tunnel: w315 -> [w507]
            tunnel: [w508] -> w316
            frame #0 {
              n203 = Greater Or Equal?(x=w507, y="Set Stress to\nComplete(Cyc/Min)") -> (x >= y?=w508:bool)
              "Stress \nCompleted(Min)" <- w507
            }
          }
          n204 = Unbundle By Name(w317) -> ("status"=w319:bool)
          n205 = call "Delay T4.vi"("milliseconds to wait"=u32 50, "error in (no error)"=w317) -> ("error out"=w330:errorcluster)  [unwired: 9 in]
          n206 = Compound Arithmetic op=OR(w316, w319, w310) -> (w297:bool)
        }
        n207 = VISA Write(VISA resource name=w246, write buffer="SOUR:FUNC VOLT;VOLT:MODE FIX;RANG 100;LEV 0.0;:SENS:FUNC \"CURR\";CURR:PROT 60E-3;RANG 100E-3;:OUTP ON", error in (no error)=w237) -> (VISA resource name out=w250:refnum<visa-resource-name>, error out=w241:errorcluster)  [unwired: 1 out]
        n208 = for {
          tunnel: w240 -> [w264]
          tunnel: w242 -> [w261] mode=indexing
          shift-right: [w259] -> w236
          shift-left: w241 -> [w265]
          tunnel: [w257] -> w239
          n209 = call "E3631A_Voltage Controller updated.vi"("VISA resource name"=w264, "I_VDD(A)"=0.2, "Channel Controller"=w261, "Voltage 1"=0.0, "Voltage 2"=3.3, "error in (no error)"=w265, "Voltage 3"=-3.3) -> ("VISA resource name out"=w257:refnum<visa-resource-name>, "error out"=w260:errorcluster)  [unwired: 7 in]
          n210 = call "Delay T4.vi"("milliseconds to wait"=u32 100, "error in (no error)"=w260) -> ("error out"=w259:errorcluster)  [unwired: 9 in]
        }
        n211 = flat-sequence {
          tunnel: w236 -> [w828]
          tunnel: [w828] -> w235
          frame #0 {
            n212 = One Button Dialog(message="Test Completed") -> ()  [unwired: 1 in, 1 out]
          }
        }
      }
      frame True {
        w830 = FALSE
      }
    }
    n213 = Wait Until Next ms Multiple(millisecond multiple=u32 100) -> ()  [unwired: 1 out]
    n214 = local write "Abort"(w57) -> ()
    n215 = local write "stop"(w58) -> ()
    n216 = Unbundle By Name(w60) -> ("status"=w75:bool)
    n217 = Compound Arithmetic op=OR(w53, w75, w67) -> (w74:bool)
    "STATUS" <- "Idle...." ("STATUS")
  }
  "Ke2000 Out" <- w24
  "PS1 Out" <- w23
  n218 = local write "Abort"(w8) -> ()
  n219 = local write "stop"(w8) -> ()
  n220 = case shown="True" w21 {
    tunnel: [w835 w837] -> w7
    tunnel: w15 -> [w835 w836]
    frame False {
    }
    frame True {
      n221 = flat-sequence {
        tunnel: w836 -> [w840]
        tunnel: [w839] -> w837
        frame #0 {
          n222 = local write "Online"(FALSE ("Online")) -> ()
          n223 = call "WSVCAP SHL Host TL Close.vi"("error in"=w840) -> ("error out"=w839:errorcluster)  [unwired: 14 in]
        }
      }
    }
  }
  "error out" <- w7
  n224 = VISA Write(VISA resource name=w16, write buffer="SOUR:FUNC VOLT;VOLT:MODE FIX;RANG 100;LEV 0.0;:SENS:FUNC \"CURR\";CURR:PROT 60E-3;RANG 100E-3;:OUTP OFF", error in (no error)=w15) -> (VISA resource name out=→"VISA resource name out":refnum<visa-resource-name>, error out=→"error out 2":errorcluster)  [unwired: 1 out]
